vi "Practica1Arduino.vi"() -> ()   [LabVIEW 2024]
uses:
  <vilib>/Instr/_visa.llb/VISA Configure Serial Port (Serial Instr).vi
panel:
  out "String":string
  in  "Boolean 2":bool
  out "Boolean":bool
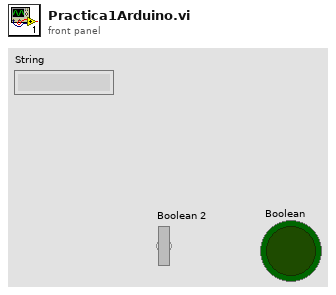
[diagram p1: front panel]
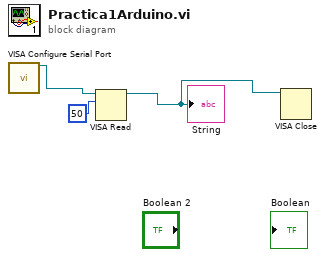
[diagram p0: block diagram]
diagram:
  n1 = call-poly "VISA Configure Serial Port"() -> ("VISA resource name out"=w3:refnum<visa-resource-name>)  [unwired: 14 in, 1 out]
  n2 = VISA Read(VISA resource name=w3, byte count=u32 50) -> (VISA resource name out=w2:refnum<visa-resource-name>)  [unwired: 1 in, 3 out]
  "String" <- w2
  n3 = VISA Close(VISA resource name=w2) -> ()  [unwired: 1 in, 1 out]
